vi "Generate Header Vectors.vi"(0 "RFFE RegWrite Command in":refnum<class "RFFE RegWrite Command.lvclass">, 11 "error in (no error)":errorcluster) -> (4 "RFFE RegWrite Command out":refnum<class "RFFE RegWrite Command.lvclass">, 6 "Header Vectors":string[](array[string]), 15 "error out":errorcluster)   [LabVIEW 2018, in "MIPI RFFE API.lvlib" / "RFFE RegWrite Command.lvclass"]
uses:
  RFFE RegWrite Command.lvclass
  C:/Users/semoore/Projects/mipi-rffe-labview-oop/Standard Command/RFFE Standard Command.lvclass
  Standard Command/RFFE Standard Command.lvclass/RFFE Standard Command.ctl
  Standard Command/Get Register Data.vi
  Standard Command/RFFE Standard Command.lvclass
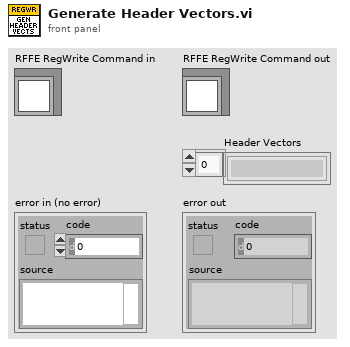
[diagram p1: front panel]
types:
  T1 = typedef "MIPI RFFE API.lvlib/Register Data.ctl" = u8
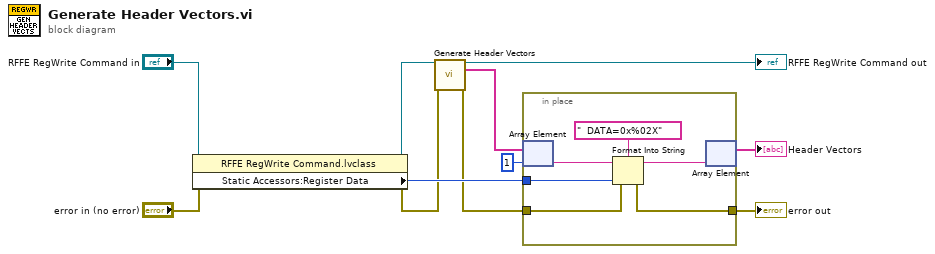
[diagram p0: block diagram]
diagram:
  n1 = property class="RFFE RegWrite Command.lvclass"(reference="RFFE RegWrite Command in", error in="error in (no error)") -> (reference out=w7:refnum<class "RFFE RegWrite Command.lvclass">, error out=w4:errorcluster, "Static Accessors:Register Data"=w9:T1)
  n2 = call-parent "Generate Header Vectors.vi"("RFFE Command in"=w7, "error in (no error)"=w4) -> ("RFFE Command out"=→"RFFE RegWrite Command out":refnum<class "RFFE RegWrite Command.lvclass">, "Header Vectors"=w11:string[], "error out"=w1:errorcluster)  [unwired: 11 in]
  n3 = in-place {
    in-place-border: w9 -> [w14]
    in-place-border: [w13] -> w2
    in-place-border: w1 -> [w12]
    n4 = in-place-array #1(w11, 1) -> (w17:string)
    n5 = Format Into String(format string="  DATA=0x%02X", initial string=w17, error in=w12, w14) -> (resulting string=w16:string, error out=w13:errorcluster)
    n6 = in-place-array #1(w16) -> (→"Header Vectors":string[])  [unwired: 1 out]
  }
  "error out" <- w2
